vi "PRL QUEUE Multiple Elements at Opposite End.vi"(8 "error in":errorcluster, 10 "Elements to Add":string[](array[string]), 11 "queue":refnum<queue>) -> (0 "error out":errorcluster, 3 "queue out":refnum<queue>)   [LabVIEW 2013, in "PMU Recorder Light.lvlib"]
uses:
  PMU Recorder Light.lvlib
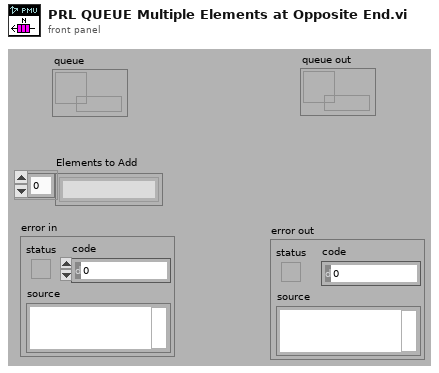
[diagram p1: front panel]
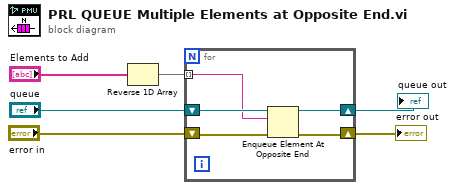
[diagram p0: block diagram]
diagram:
  n1 = Reverse 1D Array(array="Elements to Add") -> (reversed array=w2:string[])
  n2 = for {
    tunnel: w2 -> [w10] mode=indexing
    shift-right: [w8] -> w5
    shift-left: "error in" -> [w9]
    shift-right: [w7] -> w6
    shift-left: "queue" -> [w11]
    n3 = Enqueue Element At Opposite End(queue=w11, element=w10, error in (no error)=w9) -> (queue out=w7:refnum<queue>, error out=w8:errorcluster)  [unwired: 1 in, 1 out]
  }
  "error out" <- w5
  "queue out" <- w6
